vi "Write Actor Label.vi"(8 "error in (no error)":errorcluster, 10 "Actor Label":string, 11 "Monitored Actor in":refnum<class "Monitored Actor.lvclass">) -> (0 "error out":errorcluster, 3 "Monitored Actor out":refnum<class "Monitored Actor.lvclass">)   [LabVIEW 2017, in "MGI-Monitored Actor Core.lvlib" / "Monitored Actor.lvclass"]
doc: "Changes the Actor's Label. This string is displayed in the Actor Monitor window.\n----\nCopyright: MGI 2018\nAuthor: Derek Trepanier"
uses:
  Monitored Actor.lvclass
  C:/Program Files (x86)/National Instruments/LabVIEW 2017/vi.lib/ActorFramework/Actor/Actor.lvclass
  <vilib>/ActorFramework/Actor/Actor.lvclass/Actor.ctl
  <vilib>/ActorFramework/Message Enqueuer/Message Enqueuer.lvclass/Message Enqueuer.ctl
  Monitored Actor.lvclass/Monitored Actor.ctl
  <vilib>/ActorFramework/Message Enqueuer/Init from Existing Queue.vi
  <vilib>/ActorFramework/Message Enqueuer/Message Enqueuer.lvclass
  Actor Monitor/Actor Monitor Messages/Update Label Msg/Update Label Msg.lvclass
  <vilib>/ActorFramework/Actor/Actor.lvclass
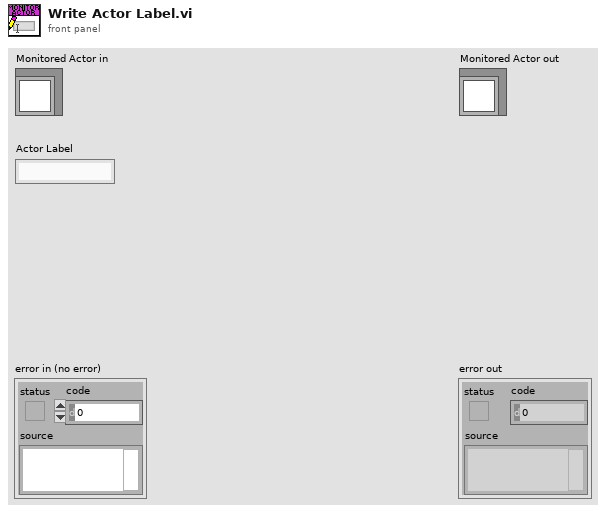
[diagram p1: front panel]
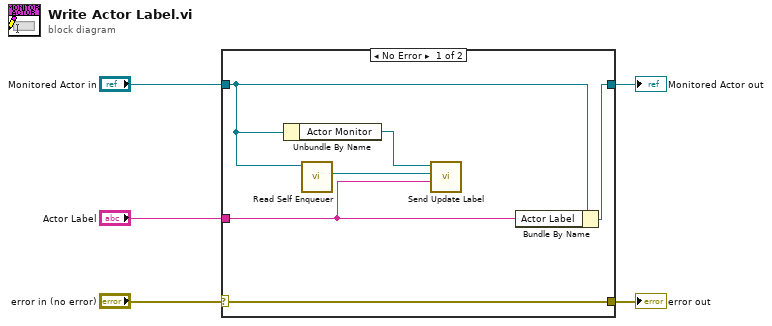
[diagram p0: block diagram]
diagram:
  n1 = case shown="No Error" "error in (no error)" {
    selector: "error in (no error)" -> [w11 w12]
    tunnel: [w11 w12] -> w4
    tunnel: [w10 w13] -> w2
    tunnel: "Monitored Actor in" -> [w9 w13]
    tunnel: "Actor Label" -> [w7 _]
    frame No Error {
      n2 = Unbundle By Name(w9) -> ("Actor Monitor"=w6:refnum<class "Message Enqueuer.lvclass">)
      n3 = call <vilib>:"Read Self Enqueuer.vi"("Actor"=w9) -> ("Self Enqueuer"=w8:refnum<class "Message Enqueuer.lvclass">)  [unwired: 10 in]
      n4 = call "Send Update Label.vi"("Actor's Label"=w7, "Actor's Self Q"=w8, "Message Enqueuer in"=w6) -> ()  [unwired: 7 in, 2 out]
      n5 = Bundle By Name(cluster=w9, "Actor Label"=w7) -> (w10:refnum<class "Monitored Actor.lvclass">)
    }
    frame Error {
    }
  }
  "error out" <- w4
  "Monitored Actor out" <- w2
